vi "Initialize.vi"(8 "Error In":errorcluster, 11 "Process In":refnum<class "Process.lvclass">) -> (0 "Error Out":errorcluster, 2 "Queue Name":string, 3 "Process Out":refnum<class "Process.lvclass">)   [LabVIEW 2019, in "Process.lvclass"]
uses:
  Process.lvclass
  Controls/Process Message.ctl
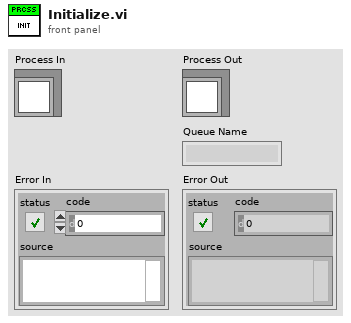
[diagram p1: front panel]
types:
  T1 = typedef "Process.lvclass/Process Message.ctl" = cluster{"Command":string, "Variant":variant}
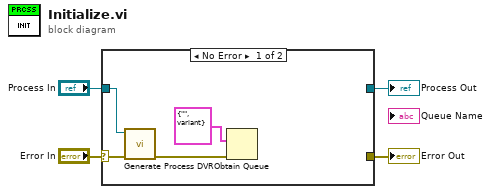
[diagram p0: block diagram]
diagram:
  n1 = case shown="No Error" "Error In" {
    selector: "Error In" -> [w7 w10]
    tunnel: [_ w10] -> w3
    tunnel: "Process In" -> [w8 w9]
    tunnel: [_ w9] -> w1
    frame No Error {
      n2 = call "Generate Process DVR.vi"("Error In"=w7, "Process In"=w8) -> ("Error Out"=w5:errorcluster)  [unwired: 8 in, 1 out]
      n3 = Obtain Queue(element data type=T1 {"Command"="", "Variant"=variant} ("Process Message"), error in (no error)=w5) -> ()  [unwired: 3 in, 3 out]
    }
    frame Error {
    }
  }
  "Process Out" <- w1
  "Error Out" <- w3
